vi "Error_manager.vi"(8 "error in (no error)":errorcluster, 10 "Caller VI":refnum<vi>, 11 "_Driver_interaction in":refnum<class "_Driver_interaction.lvclass">) -> (0 "error out":errorcluster, 1 "source":string, 2 "code":i32, 3 "_Driver_interaction out":refnum<class "_Driver_interaction.lvclass">, 5 "Step":string)   [LabVIEW 2014, in "Driver_interaction.lvlib" / "_Driver_interaction.lvclass"]
uses:
  _Driver_interaction.lvclass
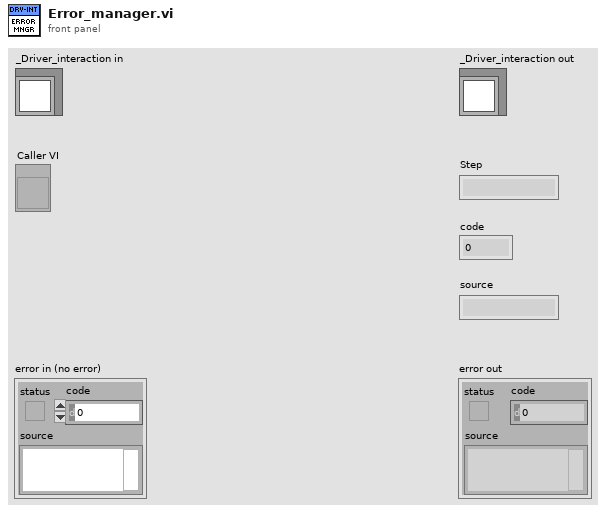
[diagram p1: front panel]
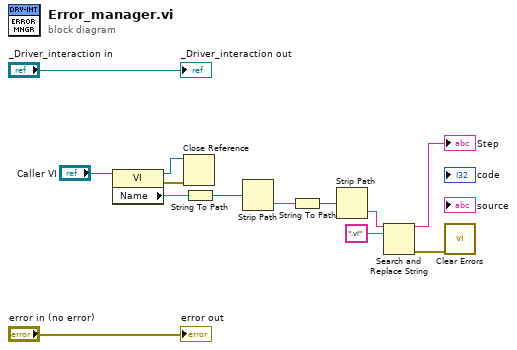
[diagram p0: block diagram]
diagram:
  n1 = property class="VI"(reference="Caller VI") -> (reference out=w11:refnum<vi>, error out=w12:errorcluster, "Name"=w10:string)  [unwired: 1 in]
  n2 = Close Reference(reference=w11, error in (no error)=w12) -> ()  [unwired: 1 out]
  n3 = String To Path(string=w10) -> (path=w9:path)
  n4 = Strip Path(path=w9) -> (name=w8:string)  [unwired: 1 out]
  n5 = String To Path(string=w8) -> (path=w7:path)
  n6 = Strip Path(path=w7) -> (name=w6:string)  [unwired: 1 out]
  n7 = Search and Replace String(input string=w6, search string=".vi") -> (result string=→"Step":string, error out=w3:errorcluster)  [unwired: 6 in, 2 out]
  n8 = call <vilib>:"Clear Errors.vi"("error in (no error)"=w3) -> ()  [unwired: 5 in, 2 out]
  "error out" <- "error in (no error)"
  "_Driver_interaction out" <- "_Driver_interaction in"
